vi "Add Key-Value Pair.vi"(8 "error in (no error)":errorcluster, 9 "value":string, 10 "key":string, 11 "URI-Component.Query in":refnum<class "URI-Component.Query.lvclass">) -> (0 "error out":errorcluster, 3 "URI-Component.Query":refnum<class "URI-Component.Query.lvclass">)   [LabVIEW 2013, in "openURI.lvlib" / "URI-Component.Query.lvclass"]
uses:
  URI-Component.Query.lvclass
  URI-Component.Query.lvclass/URI-Component.Query.ctl
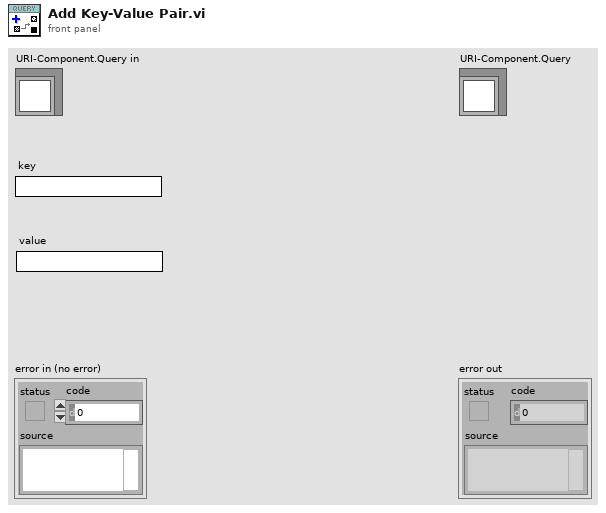
[diagram p1: front panel]
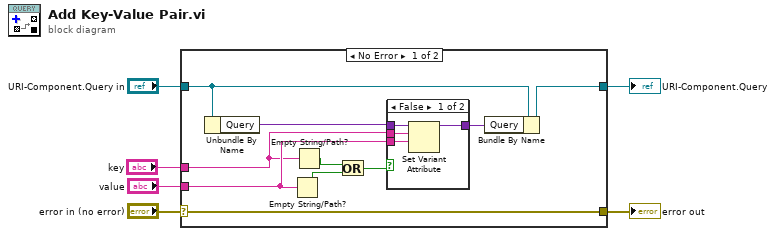
[diagram p0: block diagram]
diagram:
  n1 = case shown="No Error" "error in (no error)" {
    selector: "error in (no error)" -> [w16 w22]
    tunnel: [w16 w22] -> w5
    tunnel: [w12 w23] -> w3
    tunnel: "URI-Component.Query in" -> [w13 w23]
    tunnel: "key" -> [w10 _]
    tunnel: "value" -> [w11 _]
    frame No Error {
      n2 = Unbundle By Name(w13) -> ("Query"=w15:variant)
      n3 = Empty String/Path?(string/path=w11) -> (empty?=w8:bool)
      n4 = Empty String/Path?(string/path=w10) -> (empty?=w9:bool)
      n5 = Or(x=w9, y=w8) -> (x .or. y?=w7:bool)
      n6 = case shown="False" w7 {
        tunnel: w15 -> [w20 w21]
        tunnel: w10 -> [w19 _]
        tunnel: w11 -> [w18 _]
        tunnel: [w17 w21] -> w14
        frame False {
          n7 = Set Variant Attribute(Variant=w20, name=w19, value=w18) -> (Variant out=w17:variant)  [unwired: 1 in, 2 out]
        }
        frame True {
        }
      }
      n8 = Bundle By Name(cluster=w13, "Query"=w14) -> (w12:refnum<class "URI-Component.Query.lvclass">)
    }
    frame Error {
    }
  }
  "error out" <- w5
  "URI-Component.Query" <- w3
